vi "String to 1D Array.vi"(7 "delimiter (Tab)":string, 10 "string":string) -> (1 "Array of Strings":string[](array[string]))   [LabVIEW 2019]
doc: "Converts delimited string to a 1D array."
panel:
  # "String to 1D Array.vi - Converts delimited string to a 1D\narray.\n\nCopyright (C) 2002 James Kring jim@jimkring.com\n\nPlease visit http://www.OpenG.org to learn about the\nOpen Source LabVIEW software movement.\n\nThis library is free software; you can redistribute it and/or\nmodify it under the terms of the GNU Lesser General Public\nLicense as published by the Free Software Foundation; either\nversion 2.1 of the License, or (at your option) any later version.\nThis library is distributed in the hope that it will be useful,\nbut WITHOUT ANY WARRANTY; without even the implied warranty of\nMERCHANTABILITY or FITNESS FOR A PARTICULAR PURPOSE. See the GNU\nLesser General Public License for more details.\nYou should have received a copy of the GNU Lesser General Public\nLicense along with this library; if not, write to the Free Software\nFoundation, Inc., 59 Temple Place, Suite 330, Boston, MA 02111-1307 USA"
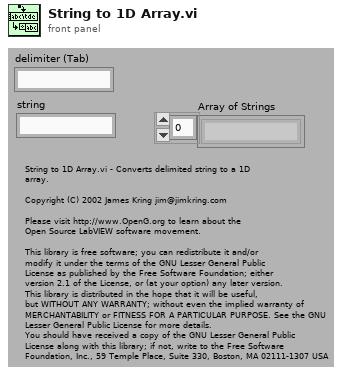
[diagram p1: front panel]
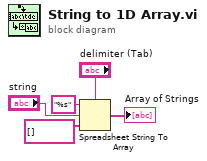
[diagram p0: block diagram]
diagram:
  n1 = Spreadsheet String To Array(delimiter (Tab)="delimiter (Tab)", format string="%s", spreadsheet string="string", array type (2D Dbl)=string[] [] ("Array Constant")) -> (array=→"Array of Strings":string[])
